vi "move.vi"(8 "error in (no error)":errorcluster, 11 "BabyHuman in":refnum<class "BabyHuman.lvclass">) -> (0 "error out":errorcluster, 2 "message":string, 3 "BabyHuman out":refnum<class "BabyHuman.lvclass">)   [LabVIEW 2017, in "BabyHuman.lvclass"]
uses:
  BabyHuman.lvclass
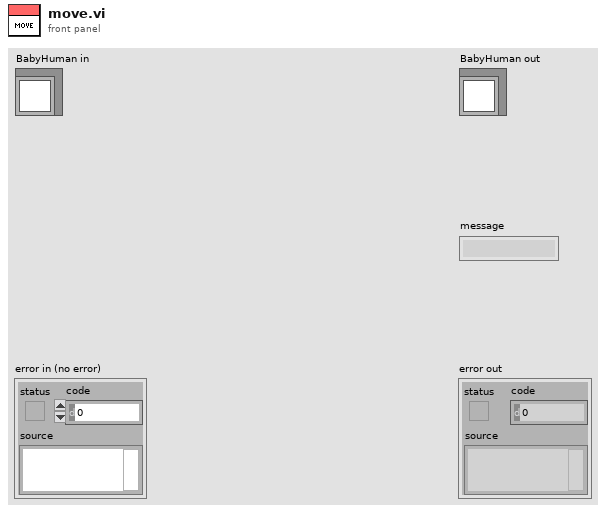
[diagram p1: front panel]
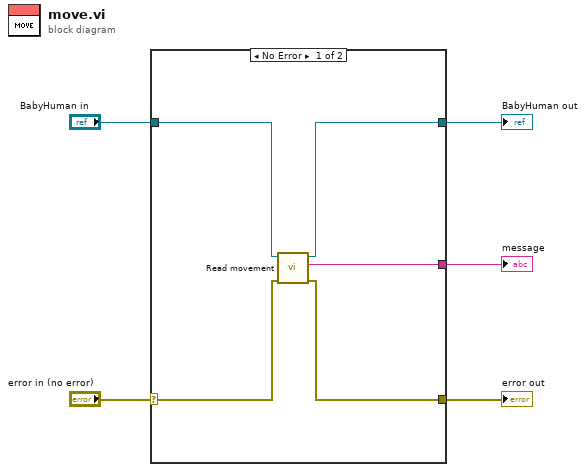
[diagram p0: block diagram]
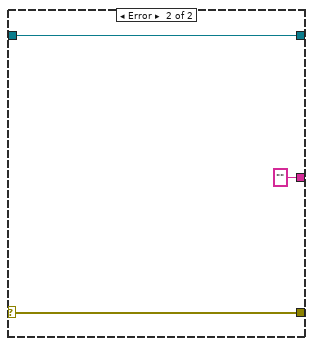
[diagram p2: hidden frame]
diagram:
  n1 = case shown="No Error" "error in (no error)" {
    selector: "error in (no error)" -> [w10 w12]
    tunnel: "BabyHuman in" -> [w8 w13]
    tunnel: [w9 w12] -> w3
    tunnel: [w7 w13] -> w2
    tunnel: [w6 "" ("movement")] -> w1
    frame No Error {
      n2 = call-dynamic "Read movement.vi"("error in (no error)"=w10, "BabyHuman in"=w8) -> ("error out"=w9:errorcluster, "movement"=w6:string, "BabyHuman out"=w7:refnum<class "BabyHuman.lvclass">)  [unwired: 7 in]
    }
    frame Error {
    }
  }
  "error out" <- w3
  "BabyHuman out" <- w2
  "message" <- w1
